vi "Array of Variants to Multi Dimensional Array Variant.vi"(7 "Dimension Lengths":i32[](array[numeric]), 8 "error in (no error)":errorcluster, 11 "[Variant]":variant[](array[variant])) -> (0 "error out":errorcluster, 3 "Array Variant":variant)   [LabVIEW 2018, in "TwinCAT ADS.lvclass"]
uses:
  TwinCAT ADS.lvclass
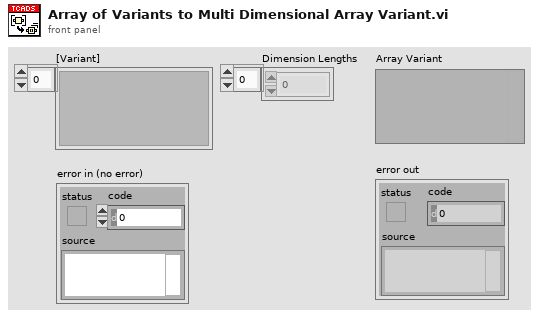
[diagram p1: front panel]
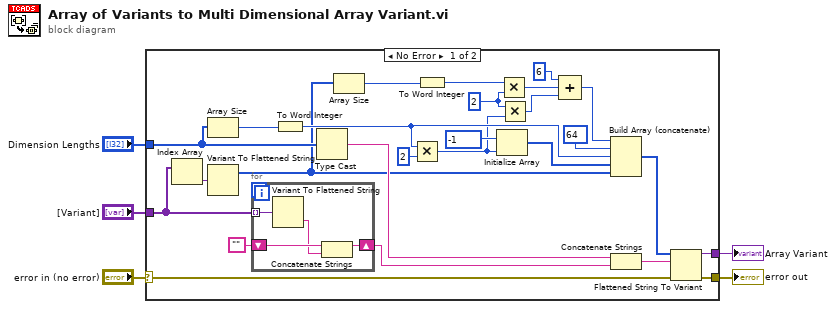
[diagram p0: block diagram]
diagram:
  n1 = case shown="No Error" "error in (no error)" {
    selector: "error in (no error)" -> [w29 w36]
    tunnel: [w28 w36] -> w4
    tunnel: "[Variant]" -> [w8 _]
    tunnel: [w27 _] -> w3
    tunnel: "Dimension Lengths" -> [w24 _]
    frame No Error {
      w13 = i16 2 ("y")
      n2 = Index Array(array=w8) -> (element=w9:variant)  [unwired: 1 in]
      n3 = Array Size(array=w24) -> (size(s)=w22:i32)
      n4 = Variant To Flattened String(Variant=w9) -> (1:w16:i16[])  [unwired: 1 out]
      n5 = for {
        tunnel: w8 -> [w35] mode=indexing
        shift-right: [w33] -> w6
        shift-left: "" -> [w34]
        n6 = Variant To Flattened String(Variant=w35) -> (data string=w32:string)  [unwired: 1 out]
        n7 = Concatenate Strings(w34, w32) -> (w33:string)
      }
      n8 = To Word Integer(number=w22) -> (16bit integer=w21:i16)
      n9 = Type Cast(x=w24) -> (*(type *) &x=w31:string)  [unwired: 1 in]
      n10 = Array Size(array=w16) -> (size(s)=w15:i32)
      n11 = Multiply(x=w21, y=i16 2) -> (x*y=w14:i16)
      n12 = To Word Integer(number=w15) -> (16bit integer=w11:i16)
      n13 = Initialize Array(i16 -1, w14) -> (w25:i16[])
      n14 = Multiply(x=w11, y=w13) -> (x*y=w17:i16)
      n15 = Multiply(x=w13, y=w14) -> (x*y=w12:i16)
      n16 = Compound Arithmetic op=ADD(i16 6 ("y"), w17, w12) -> (w18:i16)
      n17 = Build Array (concatenate)(w18, i16 64, w21, w25, w16) -> (w10:i16[])
      n18 = Concatenate Strings(w31, w6) -> (w23:string)
      n19 = Flattened String To Variant(4:w29, 6:w23, 7:w10) -> (0:w28:errorcluster, 3:w27:variant)
    }
    frame Error {
    }
  }
  "error out" <- w4
  "Array Variant" <- w3
